vi "maintenace.vi"(1 "valid":bool, 2 "Description":string, 4 "Commantaire":string, 5 "Non_technicien":string, 6 "Type maintenance":string, 7 "Durée_courroie":dbl, 8 "Error in (no error)":errorcluster, 9 "durée_huile":dbl, 10 "id":dbl, 11 "Connection In":refnum<k7>) -> (0 "Error out":errorcluster, 3 "Connection Out":refnum<k7>)   [LabVIEW 2019]
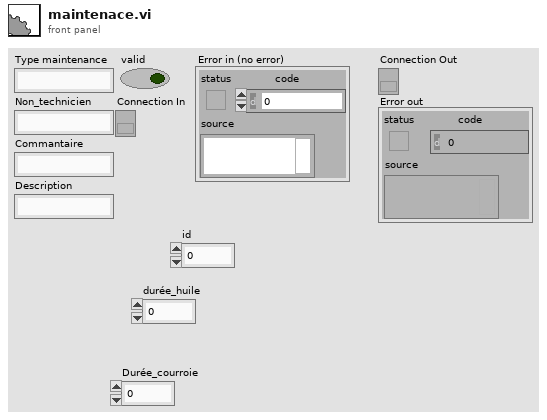
[diagram p1: front panel]
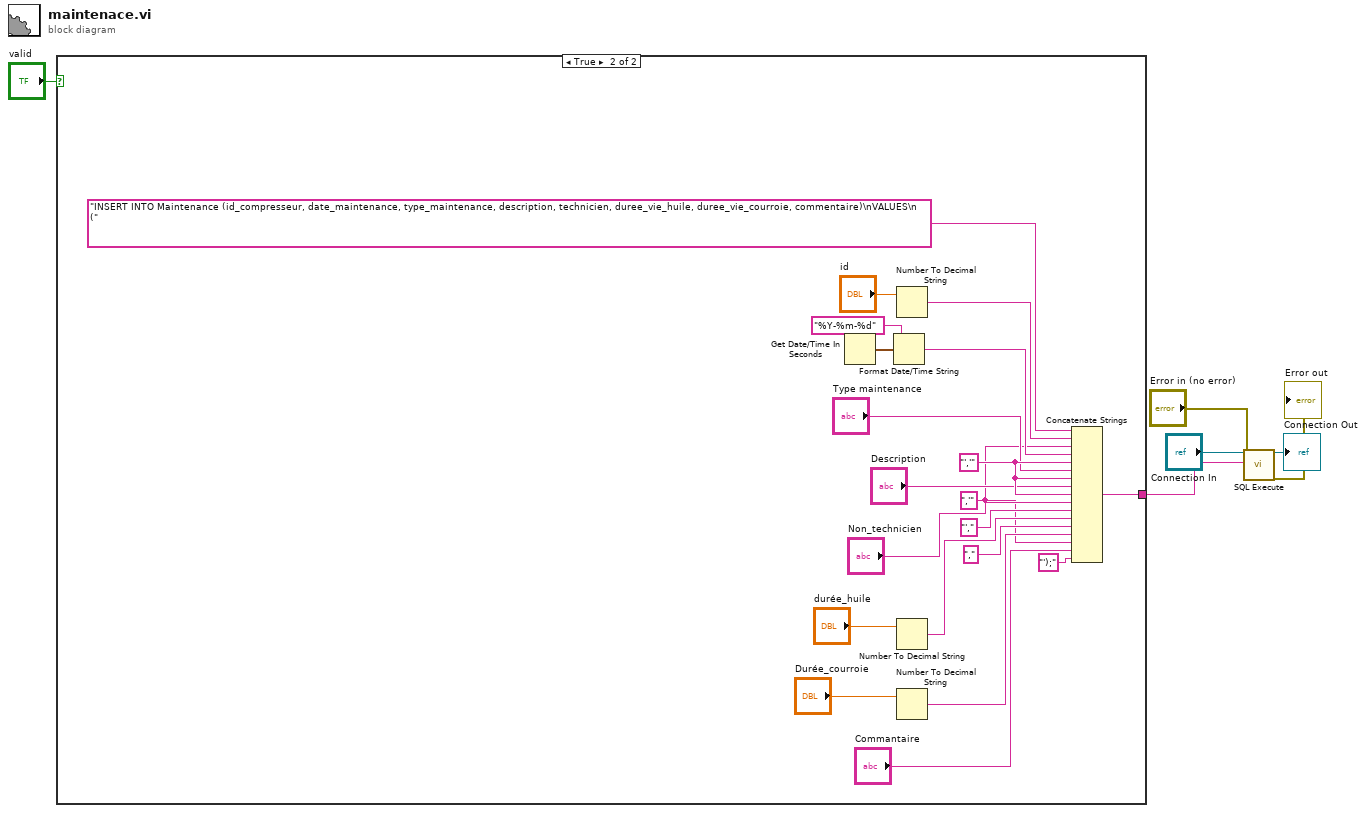
[diagram p0: block diagram]
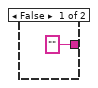
[diagram p2: hidden frame]
diagram:
  n1 = case shown="True" "valid" {
    tunnel: ["" w9] -> w6
    frame False {
    }
    frame True {
      w20 = "','" ("string")
      w12 = ",'" ("string")
      n2 = Get Date/Time In Seconds() -> (seconds since 1Jan1904=w26:timestamp)
      n3 = Format Date/Time String(time format string (%c)="%Y-%m-%d", seconds (now)=w26) -> (date/time string=w21:string)  [unwired: 1 in]
      n4 = Number To Decimal String(number="id") -> (decimal integer string=w22:string)  [unwired: 1 in]
      n5 = Number To Decimal String(number="durée_huile") -> (decimal integer string=w15:string)  [unwired: 1 in]
      n6 = Number To Decimal String(number="Durée_courroie") -> (decimal integer string=w13:string)  [unwired: 1 in]
      n7 = Concatenate Strings("INSERT INTO Maintenance (id_compresseur, date_maintenance, type_maintenance, description, technicien, duree_vie_huile, duree_vie_courroie, commentaire)\nVALUES\n    (", w22, w12, w21, w20, "Type maintenance", w20, "Description", w20, "Non_technicien", "'," ("string"), w15, "," ("string"), w13, w12, "Commantaire", "');" ("string")) -> (w9:string)
    }
  }
  n8 = call <vilib>:"SQL Execute.vi"("Connection In"="Connection In", "SQL Query"=w6, "Error in (no error)"="Error in (no error)") -> ("Connection Out"=→"Connection Out":refnum<k7>, "Error out"=→"Error out":errorcluster)  [unwired: 15 in]
